vi "POST File.vi"(6 "timeout (10000)":i32=10000, 7 "output file":path=path "", 8 "error in (no error)":errorcluster, 9 "file":path, 10 "url":string, 11 "HTTP Client Base in":refnum<class "LabVIEW HTTP Client.lvclass">) -> (0 "error out":errorcluster, 1 "body":string, 2 "headers":string, 3 "HTTP Client Base out":refnum<class "LabVIEW HTTP Client.lvclass">, 4 "status code":u32)   [LabVIEW 2020, in "HTTP Client Abstract.lvlib" / "LabVIEW HTTP Client.lvclass"]
uses:
  LabVIEW HTTP Client.lvclass
  LabVIEW HTTP Client.lvclass/LabVIEW HTTP Client.ctl
  <vilib>/httpClient/LabVIEWHTTPClient.lvlib
  Abstract HTTP Client/Abstract HTTP Client.lvclass
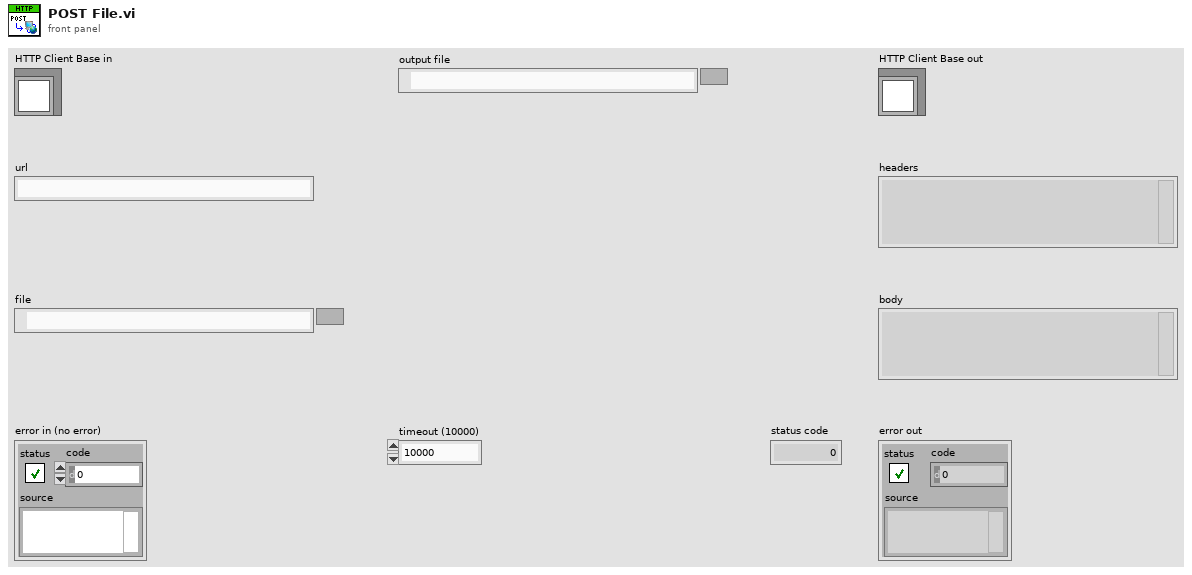
[diagram p1: front panel]
types:
  T1 = typedef "LabVIEWHTTPClient.lvlib/ClientHandle.ctl" = refnum<k1>
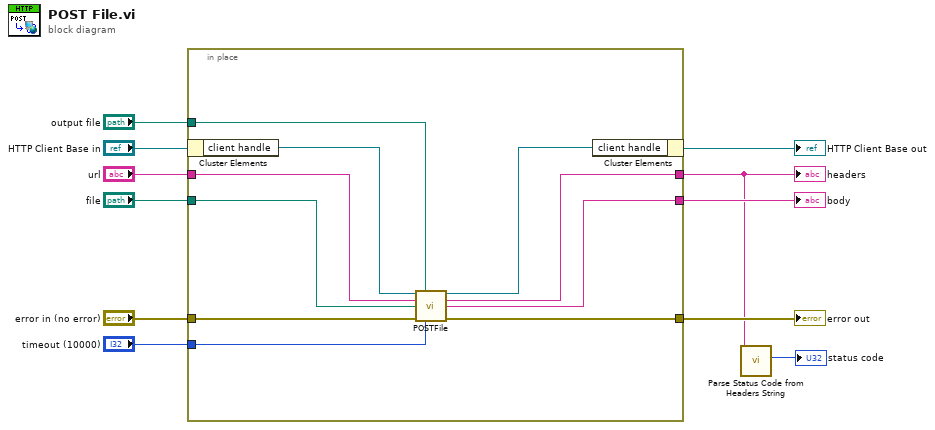
[diagram p0: block diagram]
diagram:
  n1 = in-place {
    in-place-border: "error in (no error)" -> [w21]
    in-place-border: [w20] -> w9
    in-place-border: "output file" -> [w17]
    in-place-border: "url" -> [w16]
    in-place-border: "file" -> [w15]
    in-place-border: "timeout (10000)" -> [w14]
    in-place-border: [w13] -> w1
    in-place-border: [w12] -> w3
    n2 = in-place-cluster #1("HTTP Client Base in") -> ("client handle"=w19:T1)
    n3 = call <vilib>:"POSTFile.vi"("client handle"=w19, "output file"=w17, "url"=w16, "file"=w15, "error in (no error)"=w21, "timeout (10000)"=w14) -> ("client handle out"=w18:T1, "headers"=w13:string, "body"=w12:string, "error out"=w20:errorcluster)  [unwired: 6 in]
    n4 = in-place-cluster #1("client handle"=w18) -> (→"HTTP Client Base out":refnum<class "LabVIEW HTTP Client.lvclass">)
  }
  "error out" <- w9
  "headers" <- w1
  "body" <- w3
  n5 = call "Parse Status Code from Headers String.vi"("headers in"=w1) -> ("status code"=→"status code":u32)  [unwired: 10 in]
